vi "Write Directory to create.vi"(8 "error in (no error)":errorcluster, 10 "Directory to create":string, 11 "[Test Case] Create directory in":refnum<class "[Test Case] Create directory.lvclass">) -> (0 "error out":errorcluster, 3 "[Test Case] Create directory out":refnum<class "[Test Case] Create directory.lvclass">)   [LabVIEW 2015, in "Tests.lvlib" / "[Test Case] Create directory.lvclass"]
uses:
  [Test Case] Create directory.lvclass
  [Test Case] Create directory.lvclass/[Test Case] Create directory.ctl
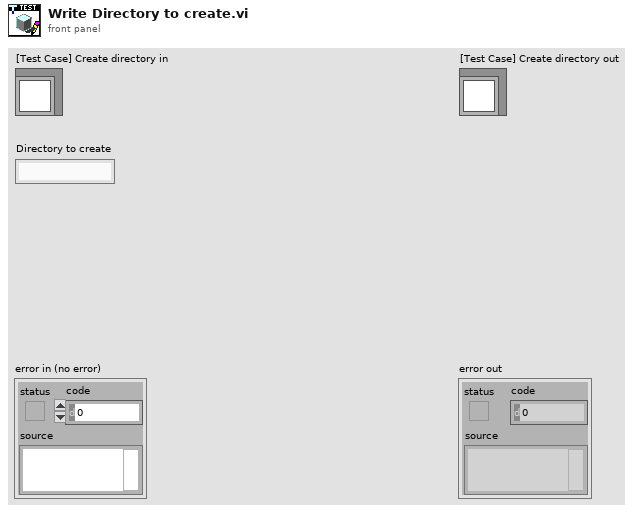
[diagram p1: front panel]
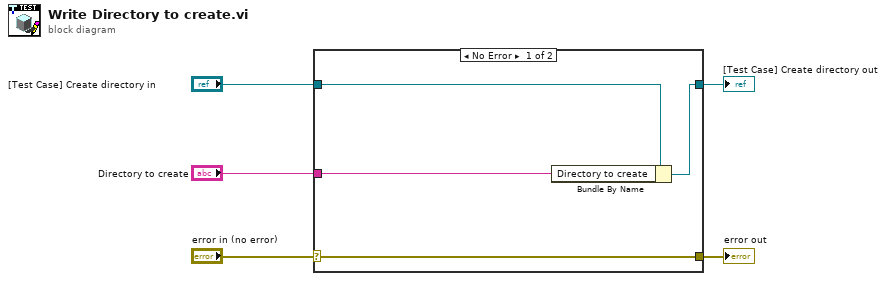
[diagram p0: block diagram]
diagram:
  n1 = case shown="No Error" "error in (no error)" {
    selector: "error in (no error)" -> [w9 w10]
    tunnel: [w9 w10] -> w4
    tunnel: [w7 w11] -> w2
    tunnel: "[Test Case] Create directory in" -> [w8 w11]
    tunnel: "Directory to create" -> [w6 _]
    frame No Error {
      n2 = Bundle By Name(cluster=w8, "Directory to create"=w6) -> (w7:refnum<class "[Test Case] Create directory.lvclass">)
    }
    frame Error {
    }
  }
  "error out" <- w4
  "[Test Case] Create directory out" <- w2
